vi "Test Reference.vi"() -> ()   [LabVIEW 2018]
panel:
  in  "Channel B Settings":T1={"Enabled"=TRUE, "Coupling"=1, "Range"=6, "Analogue Offset"=0.0} {"Range" items=["20 mV"=1, "50 mV"=2, "100 mV"=3, "200 mV"=4, "500 mV"=5, "1 V"=6, "2 V"=7, "5 V"=8, "10 V"=9, "20 V"=10]; "Coupling" items=["AC", "DC"]}
  in  "Channel A Settings":T1={"Enabled"=TRUE, "Coupling"=1, "Range"=6, "Analogue Offset"=0.0} {"Range" items=["20 mV"=1, "50 mV"=2, "100 mV"=3, "200 mV"=4, "500 mV"=5, "1 V"=6, "2 V"=7, "5 V"=8, "10 V"=9, "20 V"=10]; "Coupling" items=["AC", "DC"]}
  out "Waveform Graph 2":T2(graph)
  out "Waveform Graph":T2(graph)
  in  "Trigger Settings":T3={"Trigger Enabled"=TRUE, "Trigger Source"=enum."Channel A", "Trigger Threshold (Volts)"=0.0, "Trigger Direction"=2, "Trigger Delay (samples)"=0, "Auto Trigger Time (ms)"=1000} {"Trigger Direction" items=["Rising"=2, "Falling"=3]}
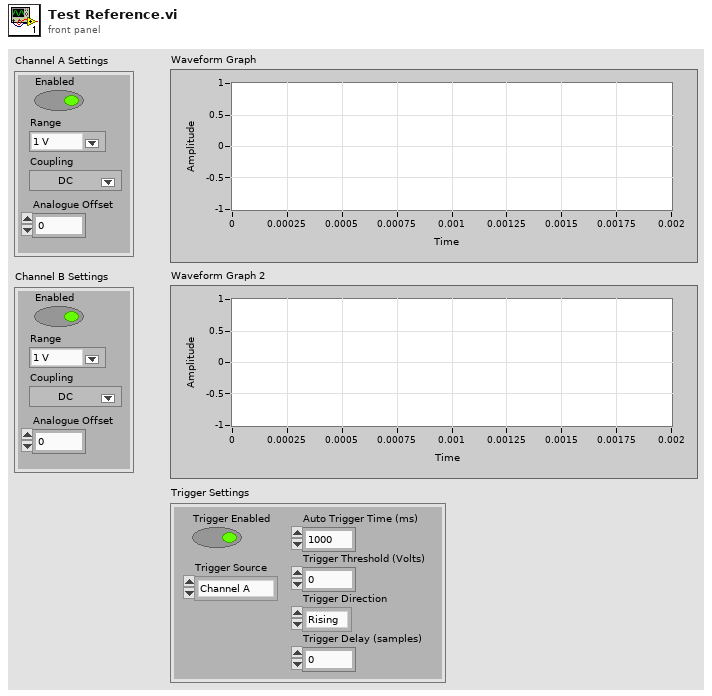
[diagram p1: front panel]
types:
  T1 = cluster{"Enabled":bool, "Coupling":i16, "Range":u16, "Analogue Offset":sgl}
  T2 = cluster{i32, "Sample Internal":sgl, "Data (Volts)":dbl[]}
  T3 = cluster{"Trigger Enabled":bool, "Trigger Source":enum16{"Channel A", "Channel B", "Channel C", "Channel D", "Ext."}, "Trigger Threshold (Volts)":dbl, "Trigger Direction":u16, "Trigger Delay (samples)":u32, "Auto Trigger Time (ms)":i16}
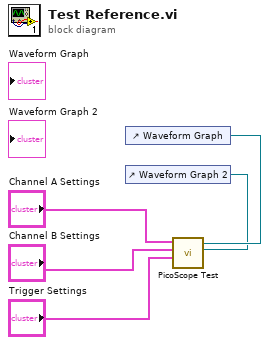
[diagram p0: block diagram]
diagram:
  n1 = control-ref of="Waveform Graph"() -> (w4:refnum<vi>)
  n2 = control-ref of="Waveform Graph 2"() -> (w3:refnum<vi>)
  n3 = call "PicoScope Test.vi"("WFD-Ref Ch-B"=w3, "WFD-Ref Ch-A"=w4, "Trigger Settings"="Trigger Settings", "Channel B Settings"="Channel B Settings", "Channel A Settings"="Channel A Settings") -> ()  [unwired: 5 in, 2 out]
